vi "Measure.vi"(8 "error in (no error)":errorcluster, 11 "Measurement in":refnum<class "Measurement.lvclass">) -> (0 "error out":errorcluster, 3 "Measurement out":refnum<class "Measurement.lvclass">)   [LabVIEW 2017, in "Measurement Actor.lvlib" / "Measurement.lvclass"]
uses:
  Measurement.lvclass
  C:/Program Files (x86)/National Instruments/LabVIEW 2017/vi.lib/ActorFramework/Actor/Actor.lvclass
  Measurement.lvclass/Measurement.ctl
  <vilib>/ActorFramework/Actor/Actor.lvclass/Actor.ctl
  <vilib>/ActorFramework/Message Enqueuer/Message Enqueuer.lvclass/Message Enqueuer.ctl
  Configuration/Step Configuration.lvclass/Step Configuration.ctl
  <vilib>/ActorFramework/Message Enqueuer/Init from Existing Queue.vi
  <vilib>/ActorFramework/Message Enqueuer/Enqueue.vi
  Messages/Acquire Msg/Acquire Msg.lvclass
  C:/Program Files (x86)/National Instruments/LabVIEW 2017/vi.lib/ActorFramework/Message/Message.lvclass
  Messages/Close Msg/Close Msg.lvclass
  <vilib>/ActorFramework/Message Priority Queue/Priority Enqueue.vi
  <vilib>/ActorFramework/Message Enqueuer/Message Enqueuer.lvclass
  Configuration/Step Configuration.lvclass
  <vilib>/ActorFramework/Actor/Actor.lvclass
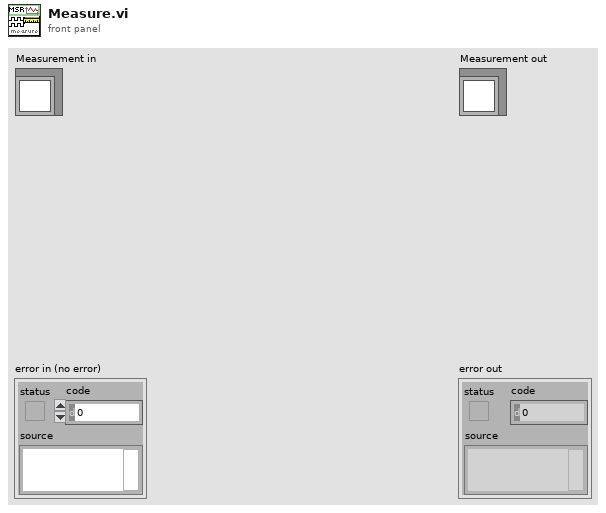
[diagram p1: front panel]
types:
  T1 = typedef "Measurement Actor.lvlib/Measurement.lvclass/Iteration count.ctl" = cluster{"Desired Iterations":i32, "Current":i32}
  T2 = cluster{"Run indefinitely":bool, "Iterations":i32}
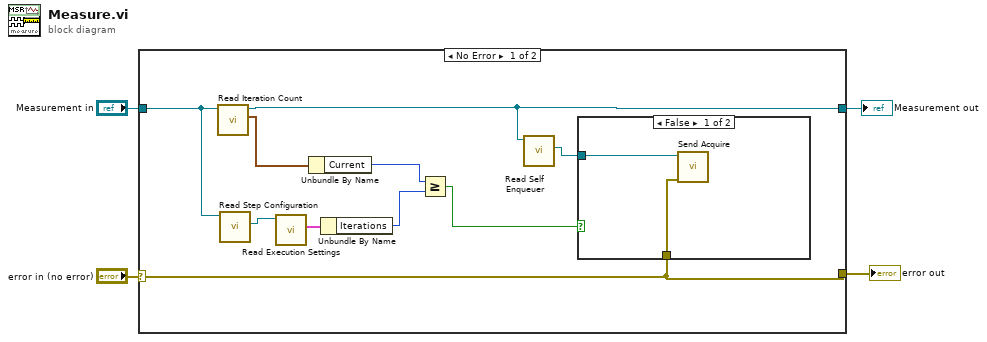
[diagram p0: block diagram]
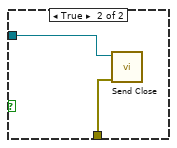
[diagram p2: hidden frame]
diagram:
  n1 = case shown="No Error" "error in (no error)" {
    selector: "error in (no error)" -> [w14 w20]
    tunnel: [w14 w20] -> w3
    tunnel: [w10 w19] -> w1
    tunnel: "Measurement in" -> [w8 w19]
    frame No Error {
      n2 = call "Read Iteration Count.vi"("Measurement in"=w8) -> ("Iteration Count"=w13:T1, "Measurement out"=w10:refnum<class "Measurement.lvclass">)  [unwired: 8 in, 1 out]
      n3 = call "Read Step Configuration.vi"("Measurement in"=w8) -> ("Measurement Actor.lvlib:Step Configuration.lvclass"=w7:refnum<class "Step Configuration.lvclass">)  [unwired: 8 in, 2 out]
      n4 = call "Read Execution Settings.vi"("Step Configuration in"=w7) -> ("Execution Settings"=w6:T2)  [unwired: 8 in, 2 out]
      n5 = Unbundle By Name(w13) -> ("Current"=w12:i32)
      n6 = Unbundle By Name(w6) -> ("Iterations"=w5:i32)
      n7 = Greater Or Equal?(x=w12, y=w5) -> (x >= y?=w11:bool)
      n8 = call <vilib>:"Read Self Enqueuer.vi"("Actor"=w10) -> ("Self Enqueuer"=w9:refnum<class "Message Enqueuer.lvclass">)  [unwired: 10 in]
      n9 = case shown="False" w11 {
        tunnel: w14 -> [w15 w18]
        tunnel: w9 -> [w16 w17]
        frame False {
          n10 = call "Send Acquire.vi"("error in (no error)"=w15, "Message Enqueuer in"=w16) -> ()  [unwired: 8 in, 2 out]
        }
        frame True {
          n11 = call "Send Close.vi"("error in (no error)"=w18, "Message Enqueuer in"=w17) -> ()  [unwired: 8 in, 2 out]
        }
      }
    }
    frame Error {
    }
  }
  "error out" <- w3
  "Measurement out" <- w1
